vi "FindPeaks.vi"(11 "subarray":cdb[](array[numeric])) -> (1 "indicies":i32[](array[numeric]))   [LabVIEW 2022 SP3]
panel:
  in  "window size":i32
  out "Array in 2":dbl[](graph)
  out "XY Graph":cluster{i32[], "Array in":dbl[]}[](graph)
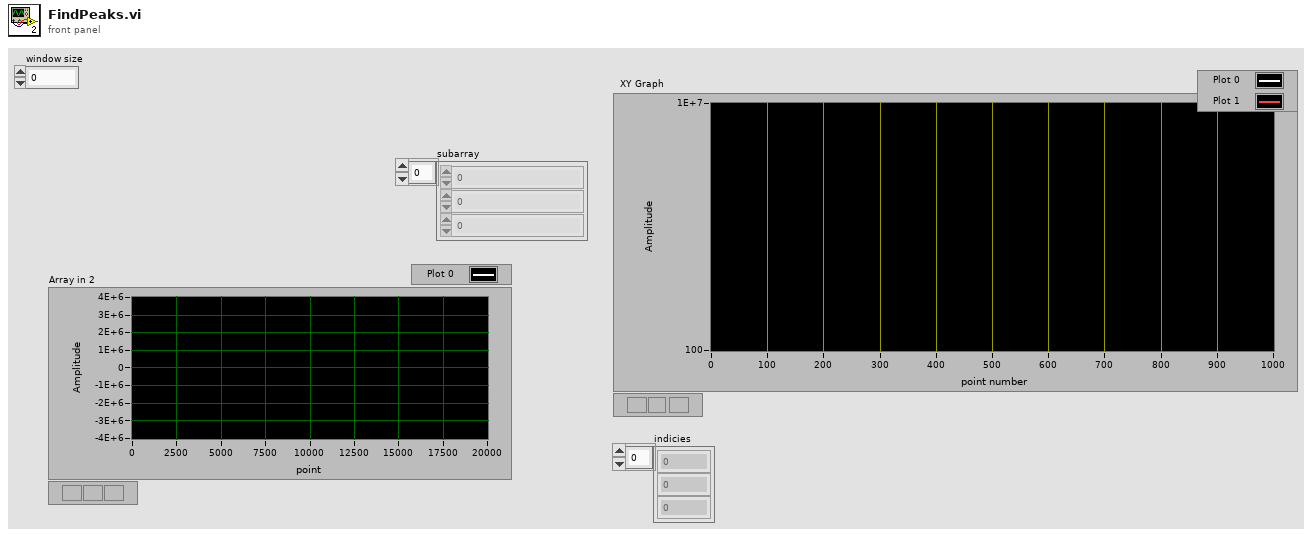
[diagram p1: front panel]
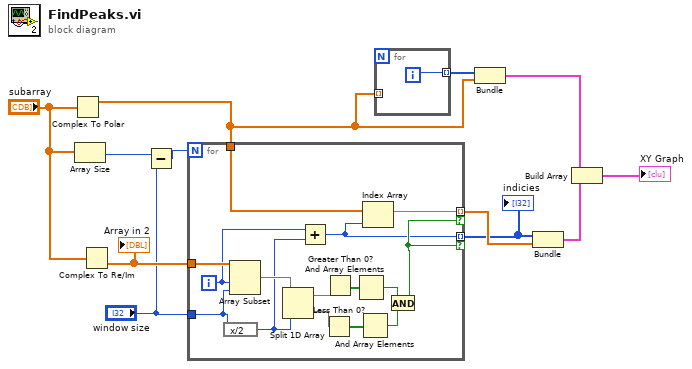
[diagram p0: block diagram]
diagram:
  n1 = Complex To Polar(r * e^(i*theta)="subarray") -> (r=w2:dbl[])  [unwired: 1 out]
  n2 = Array Size(array="subarray") -> (size(s)=w7:i32)
  n3 = Complex To Re/Im(x + iy="subarray") -> (y=w9:dbl[])  [unwired: 1 out]
  "Array in 2" <- w9
  n4 = Subtract(x=w7, y="window size") -> (x-y=w5:i32)
  n5 = for {
    N: w5 -> [_]
    tunnel: w9 -> [w19]
    tunnel: "window size" -> [w27]
    tunnel: [w13] -> w1 mode=indexing if=w18
    tunnel: [w16] -> w4 mode=indexing if=w18
    tunnel: w2 -> [w17]
    i -> [w15]
    n6 = expression code="x/2"(w27) -> (w14:i32)
    n7 = Array Subset(array=w19, index=w15, length=w27) -> (w26:dbl[])
    n8 = Split 1D Array(array=w26, index=w14) -> (first subarray=w25:dbl[], second subarray=w24:dbl[])
    n9 = Add(x=w15, y=w14) -> (x+y=w13:i32)
    n10 = Less Than 0?(x=w24) -> (x < 0?=w22:bool[])
    n11 = Greater Than 0?(x=w25) -> (x > 0?=w23:bool[])
    n12 = And Array Elements(Boolean array=w23) -> (logical AND=w21:bool)
    n13 = And Array Elements(Boolean array=w22) -> (logical AND=w20:bool)
    n14 = Index Array(array=w17, index=w13) -> (element=w16:dbl)
    n15 = And(x=w21, y=w20) -> (x .and. y?=w18:bool)
  }
  "indicies" <- w1
  n16 = for {
    tunnel: [w28] -> w12 mode=indexing
    tunnel: w2 -> [_] mode=indexing
    i -> [w28]
  }
  n17 = Bundle(w12, w2) -> (w11:cluster{i32[], dbl[]})  [unwired: 1 in]
  n18 = Bundle(w1, w4) -> (w3:cluster{i32[], dbl[]})  [unwired: 1 in]
  n19 = Build Array(w11, w3) -> (→"XY Graph":cluster{i32[], dbl[]}[])
